vi "Number to decimal string.vi"(11 "Number In":u16) -> (3 "decimal integer string out":string)   [LabVIEW 2015]
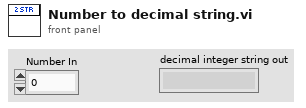
[diagram p1: front panel]
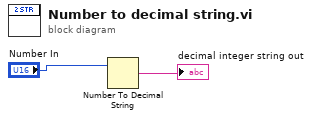
[diagram p0: block diagram]
diagram:
  n1 = Number To Decimal String(number="Number In") -> (decimal integer string=→"decimal integer string out":string)  [unwired: 1 in]
